vi "My_test.vi"(8 "VISA resource name in":refnum<visa-resource-name>) -> (0 "error out":errorcluster, 2 "Number of Bytes":u32, 3 "VISA resource name out":refnum<visa-resource-name>)   [LabVIEW 2016]
uses:
  <vilib>/Instr/_visa.llb/VISA Configure Serial Port (Instr).vi
panel:
  out "unsigned byte array":u8[](array[numeric])
  in  "error in (no error)":errorcluster
  in  "write buffer":string
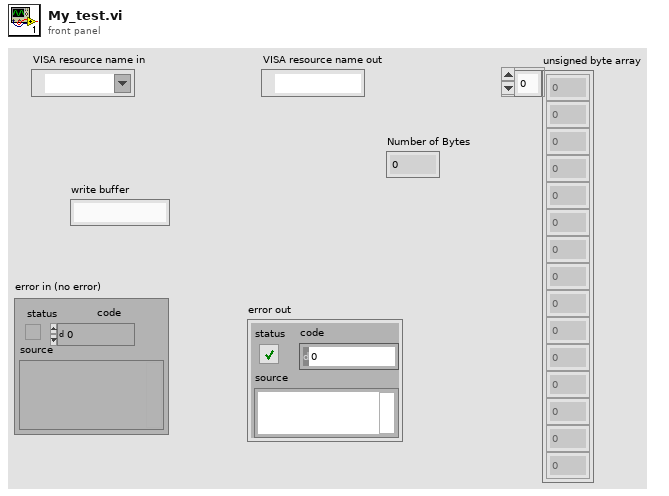
[diagram p1: front panel]
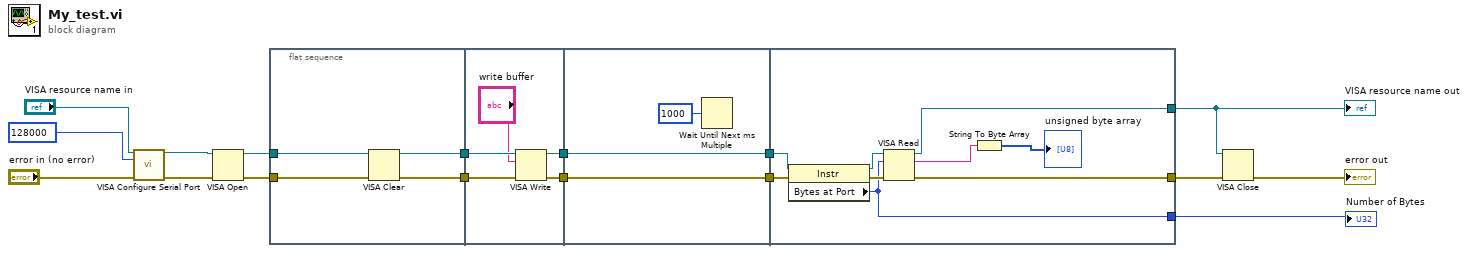
[diagram p0: block diagram]
diagram:
  n1 = call-poly "VISA Configure Serial Port"("VISA resource name"="VISA resource name in", "baud rate (9600)"=u32 128000, "error in (no error)"="error in (no error)") -> ("VISA resource name out"=w9:refnum<visa-resource-name>, "error out"=w7:errorcluster)  [unwired: 11 in]
  n2 = VISA Open(error in (no error)=w7, VISA resource name=w9) -> (VISA resource name=w5:refnum<visa-resource-name>, error out=w4:errorcluster)  [unwired: 3 in]
  n3 = flat-sequence {
    tunnel: w4 -> [w20]
    tunnel: w5 -> [w21]
    tunnel: [w19] -> w13
    tunnel: [w18] -> w12
    tunnel: [w26] -> w17
    tunnel: [w25] -> w15
    tunnel: w13 -> [w24]
    tunnel: w12 -> [w23]
    tunnel: w17 -> [w29]
    tunnel: [w29] -> w16
    tunnel: w15 -> [w28]
    tunnel: [w28] -> w14
    tunnel: w16 -> [w37]
    tunnel: [w36] -> w1
    tunnel: w14 -> [w35]
    tunnel: [w32] -> w3
    tunnel: [w33] -> w11
    frame #0 {
      n4 = VISA Clear(VISA resource name=w21, error in (no error)=w20) -> (VISA resource name out=w19:refnum<visa-resource-name>, error out=w18:errorcluster)
    }
    frame #1 {
      n5 = VISA Write(VISA resource name=w24, write buffer="write buffer", error in (no error)=w23) -> (VISA resource name out=w26:refnum<visa-resource-name>, error out=w25:errorcluster)  [unwired: 1 out]
    }
    frame #2 {
      n6 = Wait Until Next ms Multiple(millisecond multiple=u32 1000) -> ()  [unwired: 1 out]
    }
    frame #3 {
      n7 = property class="Instr"(reference=w37, error in=w35) -> (reference out=w38:refnum<visa-resource-name>, error out=w34:errorcluster, "Bytes at Port"=w33:u32)
      n8 = VISA Read(VISA resource name=w38, byte count=w33, error in (no error)=w34) -> (VISA resource name out=w36:refnum<visa-resource-name>, read buffer=w31:string, error out=w32:errorcluster)  [unwired: 1 out]
      n9 = String To Byte Array(string=w31) -> (unsigned byte array=→"unsigned byte array":u8[])
    }
  }
  n10 = VISA Close(VISA resource name=w1, error in (no error)=w3) -> (error out=→"error out":errorcluster)
  "VISA resource name out" <- w1
  "Number of Bytes" <- w11
